vi "test-swerve-drve-odometry-03.vi"() -> (3 "Test Passed":bool)   [LabVIEW 2019]
uses:
  <vilib>/Rock Robotics/WPI/ThirdParty/JAS_Junk/TrajLib/TypeDef/SWERVE_DRIVE_ODOMETRY.ctl
  <vilib>/Rock Robotics/WPI/ThirdParty/JAS_Junk/TrajLib/TypeDef/POSE2D.ctl
  <vilib>/Rock Robotics/WPI/ThirdParty/JAS_Junk/TrajLib/TypeDef/TRANSLATION2D.ctl
  <vilib>/Rock Robotics/WPI/ThirdParty/JAS_Junk/TrajLib/TypeDef/ROTATION2D.ctl
  <vilib>/Rock Robotics/WPI/ThirdParty/JAS_Junk/TrajLib/TypeDef/SWERVE_DRIVE_MODULE_POSITION.ctl
  <vilib>/Rock Robotics/WPI/ThirdParty/JAS_Junk/TrajLib/TypeDef/SWERVE_DRIVE_KINEMATICS.ctl
  <vilib>/Analysis/Matrix/Datatypes/RealMatrix.ctl
  <vilib>/Rock Robotics/WPI/ThirdParty/JAS_Junk/TrajLib/TypeDef/SWERVE_DRIVE_MODULE_STATE.ctl
  <vilib>/Rock Robotics/WPI/ThirdParty/JAS_Junk/TrajLib/Conv_Deg_Radians.vi
  <vilib>/Rock Robotics/WPI/ThirdParty/JAS_Junk/TrajLib/Rotation2d_CreateAngle.vi
  <vilib>/Rock Robotics/WPI/ThirdParty/JAS_Junk/TrajLib/Trajectory_Library.lvlib
  <vilib>/Analysis/Matrix/NI_Matrix.lvlib
panel:
  out "SWERVE_DRIVE_KINEMATICS":T1 {"SavedModuleStates"."Angle"."SIN" format="%13.4f"; "SavedModuleStates"."Angle"."COS" format="%13.4f"; "SavedModuleStates"."Angle"."VALUE" format="%13.4f"; "PrevCoR"."Y" format="%14.3f"; "PrevCoR"."X" format="%14.3f"; "Modules"."Y" format="%14.3f"; "Modules"."X" format="%14.3f"}
  out "robot POSE 3":T6={"TRANSLATION"={"X"=0.0, "Y"=0.0}, "ROTATION"={"VALUE"=0.0, "COS"=1.0, "SIN"=0.0}} {"ROTATION"."SIN" format="%13.4f"; "ROTATION"."COS" format="%13.4f"; "ROTATION"."VALUE" format="%13.4f"; "TRANSLATION"."Y" format="%14.3f"; "TRANSLATION"."X" format="%14.3f"}
  out "Odom 3":T7={"POSE"={"TRANSLATION"={"X"=0.0, "Y"=0.0}, "ROTATION"={"VALUE"=0.0, "COS"=1.0, "SIN"=0.0}}, "GyroOffset"={"VALUE"=0.0, "COS"=1.0, "SIN"=0.0}, "PreviousAngle"={"VALUE"=0.0, "COS"=1.0, "SIN"=0.0}, "PrevModulePositions"=[], "NumModules"=0} {"PrevModulePositions"."Angle"."SIN" format="%13.4f"; "PrevModulePositions"."Angle"."COS" format="%13.4f"; "PrevModulePositions"."Angle"."VALUE" format="%13.4f"; "PreviousAngle"."SIN" format="%13.4f"; "PreviousAngle"."COS" format="%13.4f"; "PreviousAngle"."VALUE" format="%13.4f"; "GyroOffset"."SIN" format="%13.4f"; "GyroOffset"."COS" format="%13.4f"; "GyroOffset"."VALUE" format="%13.4f"; "POSE"."ROTATION"."SIN" format="%13.4f"; "POSE"."ROTATION"."COS" format="%13.4f"; "POSE"."ROTATION"."VALUE" format="%13.4f"; "POSE"."TRANSLATION"."Y" format="%14.3f"; "POSE"."TRANSLATION"."X" format="%14.3f"}
  out "Odom 1":T7={"POSE"={"TRANSLATION"={"X"=0.0, "Y"=0.0}, "ROTATION"={"VALUE"=0.0, "COS"=1.0, "SIN"=0.0}}, "GyroOffset"={"VALUE"=0.0, "COS"=1.0, "SIN"=0.0}, "PreviousAngle"={"VALUE"=0.0, "COS"=1.0, "SIN"=0.0}, "PrevModulePositions"=[], "NumModules"=0} {"PrevModulePositions"."Angle"."SIN" format="%13.4f"; "PrevModulePositions"."Angle"."COS" format="%13.4f"; "PrevModulePositions"."Angle"."VALUE" format="%13.4f"; "PreviousAngle"."SIN" format="%13.4f"; "PreviousAngle"."COS" format="%13.4f"; "PreviousAngle"."VALUE" format="%13.4f"; "GyroOffset"."SIN" format="%13.4f"; "GyroOffset"."COS" format="%13.4f"; "GyroOffset"."VALUE" format="%13.4f"; "POSE"."ROTATION"."SIN" format="%13.4f"; "POSE"."ROTATION"."COS" format="%13.4f"; "POSE"."ROTATION"."VALUE" format="%13.4f"; "POSE"."TRANSLATION"."Y" format="%14.3f"; "POSE"."TRANSLATION"."X" format="%14.3f"}
  out "Odom 0":T7={"POSE"={"TRANSLATION"={"X"=0.0, "Y"=0.0}, "ROTATION"={"VALUE"=0.0, "COS"=1.0, "SIN"=0.0}}, "GyroOffset"={"VALUE"=0.0, "COS"=1.0, "SIN"=0.0}, "PreviousAngle"={"VALUE"=0.0, "COS"=1.0, "SIN"=0.0}, "PrevModulePositions"=[], "NumModules"=0} {"PrevModulePositions"."Angle"."SIN" format="%13.4f"; "PrevModulePositions"."Angle"."COS" format="%13.4f"; "PrevModulePositions"."Angle"."VALUE" format="%13.4f"; "PreviousAngle"."SIN" format="%13.4f"; "PreviousAngle"."COS" format="%13.4f"; "PreviousAngle"."VALUE" format="%13.4f"; "GyroOffset"."SIN" format="%13.4f"; "GyroOffset"."COS" format="%13.4f"; "GyroOffset"."VALUE" format="%13.4f"; "POSE"."ROTATION"."SIN" format="%13.4f"; "POSE"."ROTATION"."COS" format="%13.4f"; "POSE"."ROTATION"."VALUE" format="%13.4f"; "POSE"."TRANSLATION"."Y" format="%14.3f"; "POSE"."TRANSLATION"."X" format="%14.3f"}
  out "robot POSE 0":T6={"TRANSLATION"={"X"=0.0, "Y"=0.0}, "ROTATION"={"VALUE"=0.0, "COS"=1.0, "SIN"=0.0}} {"ROTATION"."SIN" format="%13.4f"; "ROTATION"."COS" format="%13.4f"; "ROTATION"."VALUE" format="%13.4f"; "TRANSLATION"."Y" format="%14.3f"; "TRANSLATION"."X" format="%14.3f"}
  out "robot POSE 2":T6={"TRANSLATION"={"X"=0.0, "Y"=0.0}, "ROTATION"={"VALUE"=0.0, "COS"=1.0, "SIN"=0.0}} {"ROTATION"."SIN" format="%13.4f"; "ROTATION"."COS" format="%13.4f"; "ROTATION"."VALUE" format="%13.4f"; "TRANSLATION"."Y" format="%14.3f"; "TRANSLATION"."X" format="%14.3f"}
  out "Odom 2":T7={"POSE"={"TRANSLATION"={"X"=0.0, "Y"=0.0}, "ROTATION"={"VALUE"=0.0, "COS"=1.0, "SIN"=0.0}}, "GyroOffset"={"VALUE"=0.0, "COS"=1.0, "SIN"=0.0}, "PreviousAngle"={"VALUE"=0.0, "COS"=1.0, "SIN"=0.0}, "PrevModulePositions"=[], "NumModules"=0} {"PrevModulePositions"."Angle"."SIN" format="%13.4f"; "PrevModulePositions"."Angle"."COS" format="%13.4f"; "PrevModulePositions"."Angle"."VALUE" format="%13.4f"; "PreviousAngle"."SIN" format="%13.4f"; "PreviousAngle"."COS" format="%13.4f"; "PreviousAngle"."VALUE" format="%13.4f"; "GyroOffset"."SIN" format="%13.4f"; "GyroOffset"."COS" format="%13.4f"; "GyroOffset"."VALUE" format="%13.4f"; "POSE"."ROTATION"."SIN" format="%13.4f"; "POSE"."ROTATION"."COS" format="%13.4f"; "POSE"."ROTATION"."VALUE" format="%13.4f"; "POSE"."TRANSLATION"."Y" format="%14.3f"; "POSE"."TRANSLATION"."X" format="%14.3f"}
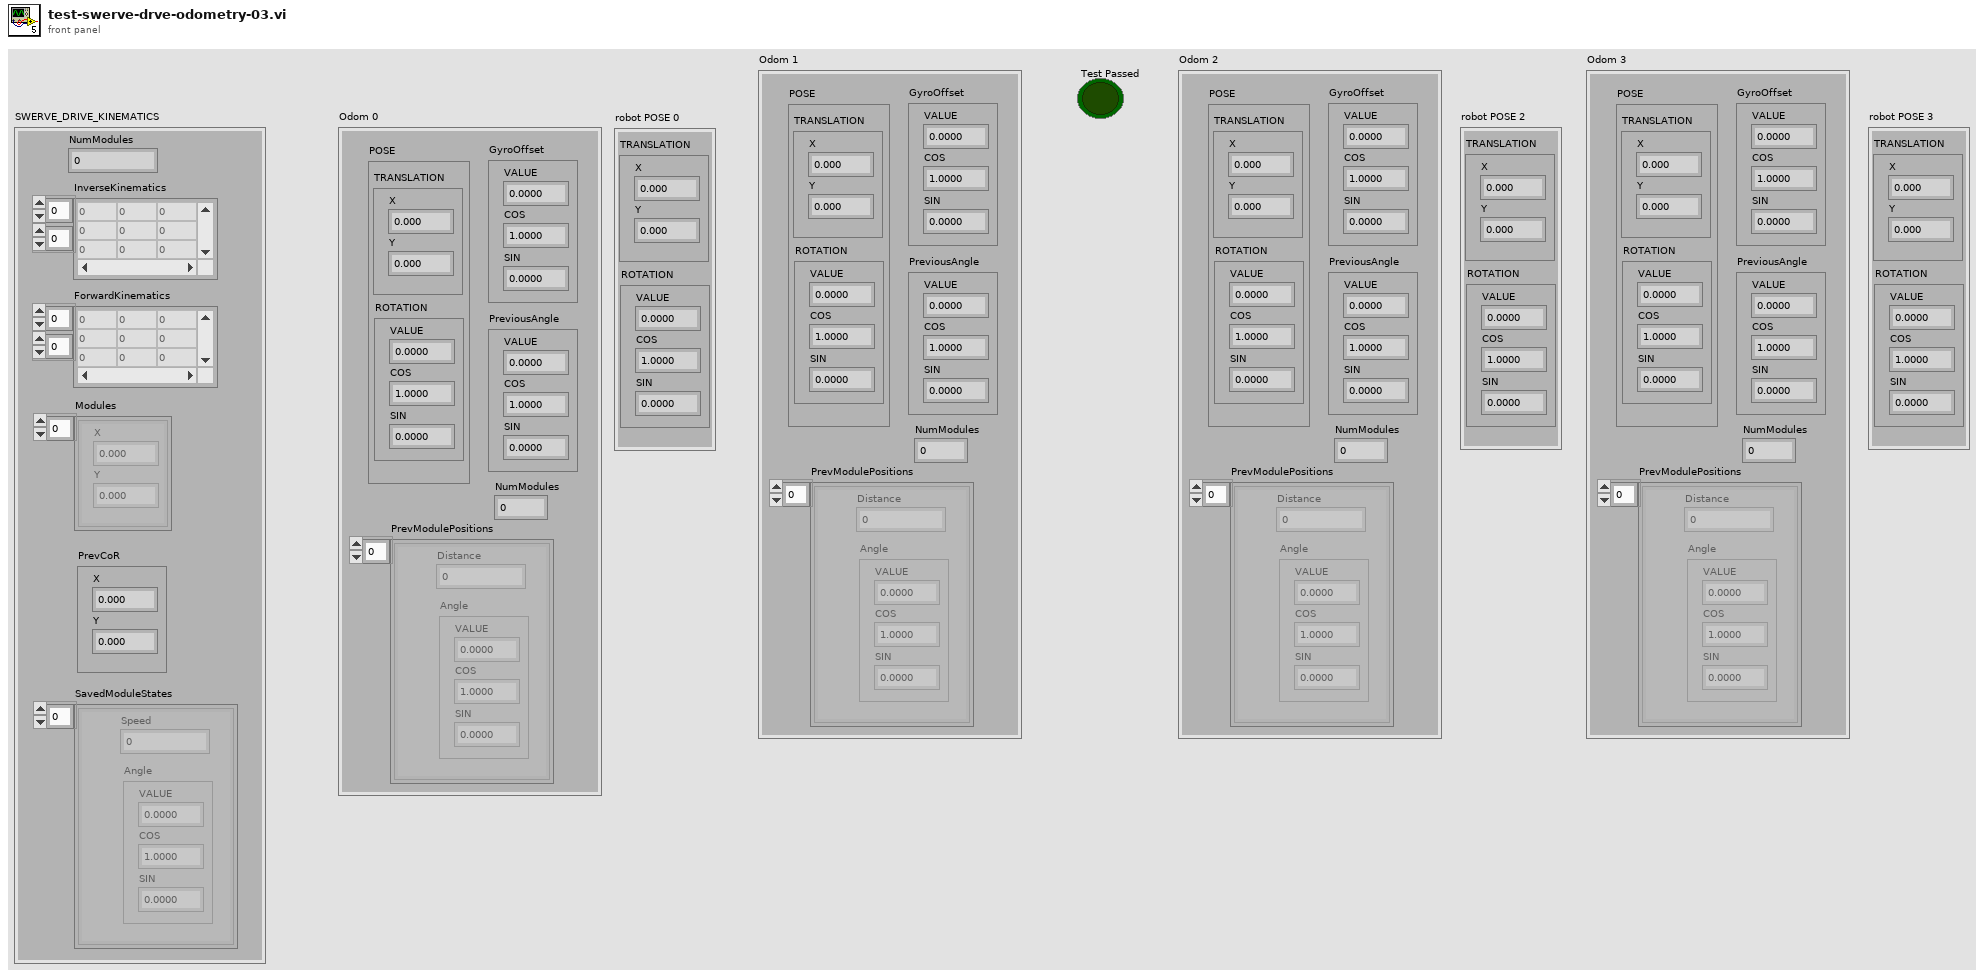
[diagram p1: front panel]
types:
  T1 = typedef "Trajectory_Library.lvlib/SWERVE_DRIVE_KINEMATICS.ctl" = cluster{"NumModules":i32, "InverseKinematics":T2, "ForwardKinematics":T2, "Modules":T3[], "PrevCoR":T3, "SavedModuleStates":T4[]}
  T2 = typedef "NI_Matrix.lvlib/RealMatrix.ctl" = dbl[][]
  T3 = typedef "Trajectory_Library.lvlib/TRANSLATION2D.ctl" = cluster{"X":dbl, "Y":dbl}
  T4 = typedef "Trajectory_Library.lvlib/SWERVE_DRIVE_MODULE_STATE.ctl" = cluster{"Speed":dbl, "Angle":T5}
  T5 = typedef "Trajectory_Library.lvlib/ROTATION2D.ctl" = cluster{"VALUE":dbl, "COS":dbl, "SIN":dbl}
  T6 = typedef "Trajectory_Library.lvlib/POSE2D.ctl" = cluster{"TRANSLATION":T3, "ROTATION":T5}
  T7 = typedef "Trajectory_Library.lvlib/SWERVE_DRIVE_ODOMETRY.ctl" = cluster{"POSE":T6, "GyroOffset":T5, "PreviousAngle":T5, "PrevModulePositions":T8[], "NumModules":i32}
  T8 = typedef "Trajectory_Library.lvlib/SWERVE_DRIVE_MODULE_POSITION.ctl" = cluster{"Distance":dbl, "Angle":T5}
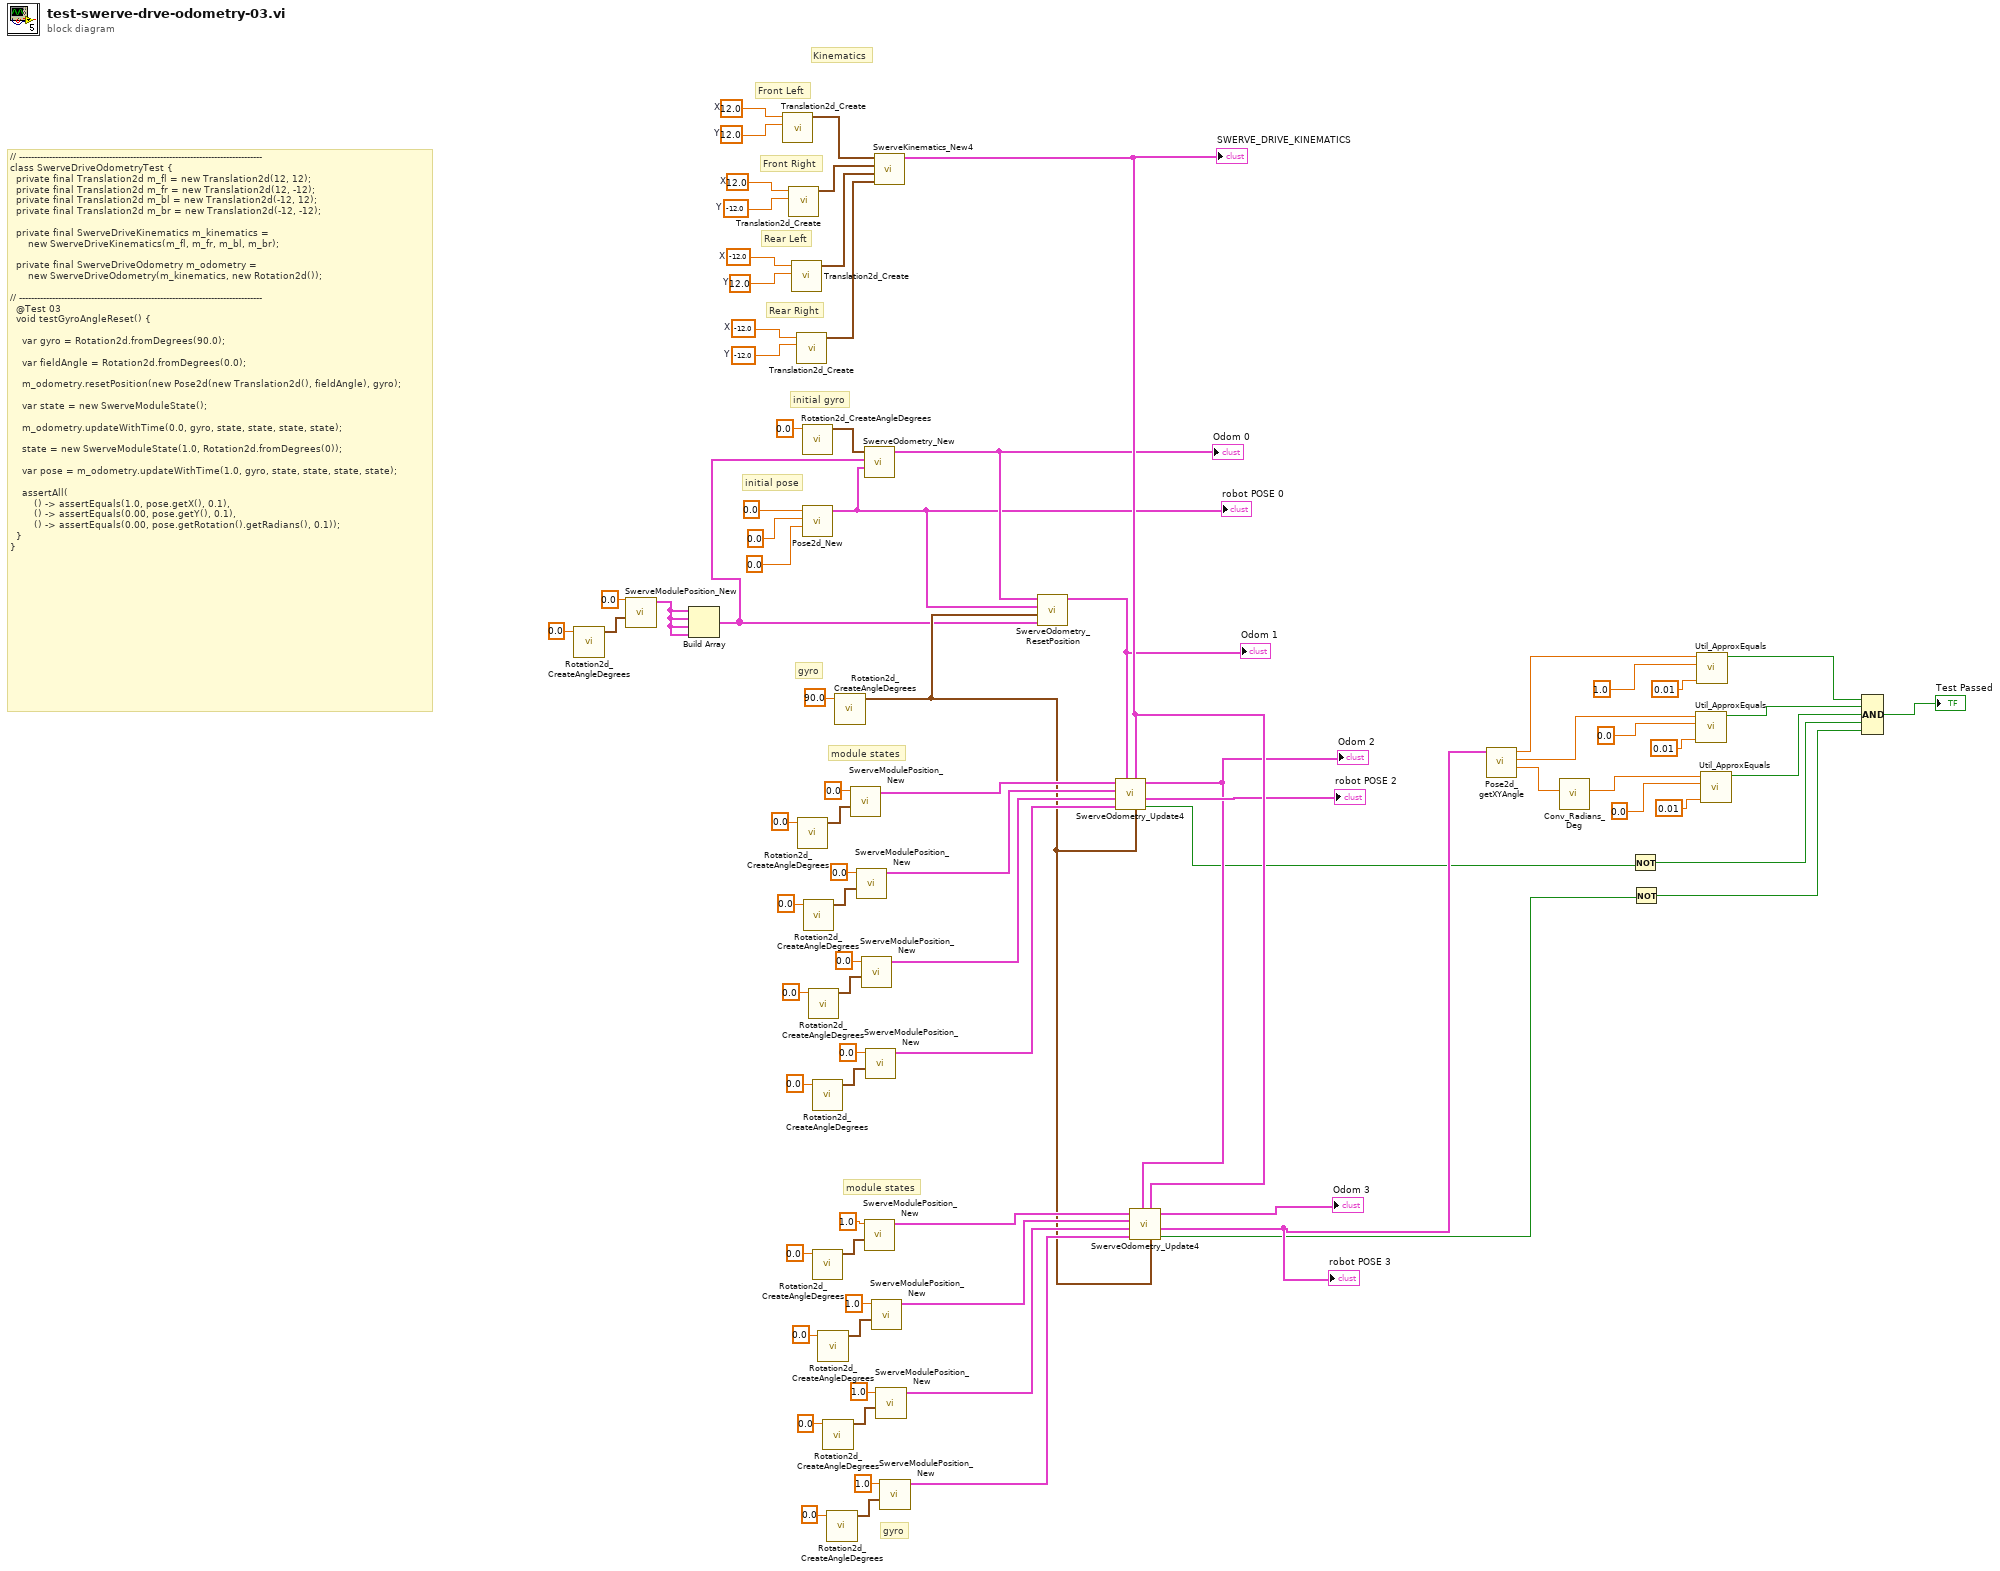
[diagram p0: block diagram]
diagram:
  w78 = -12.0  # X
  w77 = -12.0  # Y
  w76 = -12.0  # X
  w75 = 12.0  # Y
  w74 = 12.0  # X
  w73 = -12.0  # Y
  w72 = 12.0  # X
  w71 = 12.0  # Y
  # "gyro"
  # "initial pose"
  # "gyro"
  # "module states"
  # "module states"
  # "Kinematics"
  # "initial gyro"
  # "Rear Right"
  # "Rear Left"
  # "Front Right"
  # "Front Left"
  # "// ---------------------------------------------------------------------------------\nclass SwerveDriveOdometryTest {\n  private final Translation2d m_fl = new Translation2d(12, 12);\n  private final Translation2d m_fr = new Translation2d(12, -12);\n  private final Translation2d m_bl = new Translation2d(-12, 12);\n  private final Translation2d m_br = new Translation2d(-12, -12);\n\n  private final SwerveDriveKinematics m_kinematics =\n      new SwerveDriveKinematics(m_fl, m_fr, m_bl, m_br);\n\n  private final SwerveDriveOdometry m_odometry =\n      new SwerveDriveOdometry(m_kinematics, new Rotation2d());\n\n// ---------------------------------------------------------------------------------\n  @Test 03\n  void testGyroAngleReset() {\n\n    var gyro = Rotation2d.fromDegrees(90.0);\n\n    var fieldAngle = Rotation2d.fromDegrees(0.0);\n\n    m_odometry.resetPosition(new Pose2d(new Translation2d(), fieldAngle), gyro);\n\n    var state = new SwerveModuleState();\n\n    m_odometry.updateWithTime(0.0, gyro, state, state, state, state);\n\n    state = new SwerveModuleState(1.0, Rotation2d.fromDegrees(0));\n\n    var pose = m_odometry.updateWithTime(1.0, gyro, state, state, state, state);\n\n    assertAll(\n        () -> assertEquals(1.0, pose.getX(), 0.1),\n        () -> assertEquals(0.00, pose.getY(), 0.1),\n        () -> assertEquals(0.00, pose.getRotation().getRadians(), 0.1));\n  }\n}"
  n1 = call <vilib>:"Rotation2d_CreateAngleDegrees.vi"("Angle_Degrees"=0.0) -> ("ROTATION"=w8:T5)  [unwired: 10 in]
  n2 = call <vilib>:"SwerveModulePosition_New.vi"("ROTATION"=w8, "Distance"=0.0 ("Speed")) -> ("SWERVE_DRIVE_MODULE_POSITION"=w6:T8)  [unwired: 9 in]
  n3 = Build Array(w6, w6, w6, w6) -> (w5:T8[])
  n4 = call <vilib>:"Translation2d_Create.vi"("Y"=w71, "X"=w72) -> ("TRANSLATION"=w79:T3)  [unwired: 9 in]
  n5 = call <vilib>:"Translation2d_Create.vi"("Y"=w73, "X"=w74) -> ("TRANSLATION"=w80:T3)  [unwired: 9 in]
  n6 = call <vilib>:"Translation2d_Create.vi"("Y"=w75, "X"=w76) -> ("TRANSLATION"=w81:T3)  [unwired: 9 in]
  n7 = call <vilib>:"Translation2d_Create.vi"("Y"=w77, "X"=w78) -> ("TRANSLATION"=w82:T3)  [unwired: 9 in]
  n8 = call <vilib>:"Rotation2d_CreateAngleDegrees.vi"("Angle_Degrees"=0.0) -> ("ROTATION"=w64:T5)  [unwired: 10 in]
  n9 = call <vilib>:"Rotation2d_CreateAngleDegrees.vi"("Angle_Degrees"=0.0) -> ("ROTATION"=w67:T5)  [unwired: 10 in]
  n10 = call <vilib>:"Pose2d_New.vi"("Heading"=0.0, "Y"=0.0, "X"=0.0) -> ("out POSe"=w13:T6)  [unwired: 8 in]
  "robot POSE 0" <- w13
  n11 = call <vilib>:"Rotation2d_CreateAngleDegrees.vi"("Angle_Degrees"=0.0) -> ("ROTATION"=w61:T5)  [unwired: 10 in]
  n12 = call <vilib>:"Rotation2d_CreateAngleDegrees.vi"("Angle_Degrees"=0.0) -> ("ROTATION"=w58:T5)  [unwired: 10 in]
  n13 = call <vilib>:"Rotation2d_CreateAngleDegrees.vi"("Angle_Degrees"=0.0) -> ("ROTATION"=w55:T5)  [unwired: 10 in]
  n14 = call <vilib>:"Rotation2d_CreateAngleDegrees.vi"("Angle_Degrees"=0.0) -> ("ROTATION"=w48:T5)  [unwired: 10 in]
  n15 = call <vilib>:"Rotation2d_CreateAngleDegrees.vi"("Angle_Degrees"=0.0) -> ("ROTATION"=w45:T5)  [unwired: 10 in]
  n16 = call <vilib>:"Rotation2d_CreateAngleDegrees.vi"("Angle_Degrees"=0.0) -> ("ROTATION"=w42:T5)  [unwired: 10 in]
  n17 = call <vilib>:"Rotation2d_CreateAngleDegrees.vi"("Angle_Degrees"=0.0) -> ("ROTATION"=w39:T5)  [unwired: 10 in]
  n18 = call <vilib>:"Rotation2d_CreateAngleDegrees.vi"("Angle_Degrees"=90.0) -> ("ROTATION"=w12:T5)  [unwired: 10 in]
  n19 = call <vilib>:"SwerveModulePosition_New.vi"("ROTATION"=w64, "Distance"=0.0 ("Speed")) -> ("SWERVE_DRIVE_MODULE_POSITION"=w53:T8)  [unwired: 9 in]
  n20 = call <vilib>:"SwerveModulePosition_New.vi"("ROTATION"=w61, "Distance"=0.0 ("Speed")) -> ("SWERVE_DRIVE_MODULE_POSITION"=w52:T8)  [unwired: 9 in]
  n21 = call <vilib>:"SwerveModulePosition_New.vi"("ROTATION"=w58, "Distance"=0.0 ("Speed")) -> ("SWERVE_DRIVE_MODULE_POSITION"=w51:T8)  [unwired: 9 in]
  n22 = call <vilib>:"SwerveOdometry_New.vi"("InitialPose"=w13, "Module Positions"=w5, "gyroAngle"=w67) -> ("SWERVE_DRIVE_ODOMETRY"=w18:T7)  [unwired: 8 in]
  "Odom 0" <- w18
  n23 = call <vilib>:"SwerveModulePosition_New.vi"("ROTATION"=w48, "Distance"=1.0 ("Speed")) -> ("SWERVE_DRIVE_MODULE_POSITION"=w37:T8)  [unwired: 9 in]
  n24 = call <vilib>:"SwerveModulePosition_New.vi"("ROTATION"=w55, "Distance"=0.0 ("Speed")) -> ("SWERVE_DRIVE_MODULE_POSITION"=w50:T8)  [unwired: 9 in]
  n25 = call <vilib>:"SwerveModulePosition_New.vi"("ROTATION"=w45, "Distance"=1.0 ("Speed")) -> ("SWERVE_DRIVE_MODULE_POSITION"=w36:T8)  [unwired: 9 in]
  n26 = call <vilib>:"SwerveKinematics_New4.vi"("wheel 3"=w82, "wheel 2"=w81, "wheel 1"=w80, "wheel 0"=w79) -> ("SWERVE_DRIVE_KINEMATICS"=w33:T1)  [unwired: 7 in]
  "SWERVE_DRIVE_KINEMATICS" <- w33
  n27 = call <vilib>:"SwerveModulePosition_New.vi"("ROTATION"=w42, "Distance"=1.0 ("Speed")) -> ("SWERVE_DRIVE_MODULE_POSITION"=w35:T8)  [unwired: 9 in]
  n28 = call <vilib>:"SwerveModulePosition_New.vi"("ROTATION"=w39, "Distance"=1.0 ("Speed")) -> ("SWERVE_DRIVE_MODULE_POSITION"=w34:T8)  [unwired: 9 in]
  n29 = call <vilib>:"SwerveOdometry_ResetPosition.vi"("Module Positions"=w5, "gyroAngle"=w12, "Pose"=w13, "in SWERVE_DRIVE_ODOMETRY"=w18) -> ("out SWERVE_DRIVE_ODOMETRY"=w17:T7)  [unwired: 6 in, 1 out]
  "Odom 1" <- w17
  n30 = call <vilib>:"SwerveOdometry_Update4.vi"("gyroAngle"=w12, "SWERVE_DRIVE_KINEMATICS"=w33, "in SWERVE_DRIVE_ODOMETRY"=w17, "Wheel Position 3"=w50, "Wheel Position 2"=w51, "Wheel Position 1"=w52, "Wheel Position 0"=w53) -> ("Error"=w4:bool, "robot POSE"=→"robot POSE 2":T6, "out SWERVE_DRIVE_ODOMETRY"=w15:T7)  [unwired: 2 in]
  "Odom 2" <- w15
  n31 = call <vilib>:"SwerveOdometry_Update4.vi"("gyroAngle"=w12, "SWERVE_DRIVE_KINEMATICS"=w33, "in SWERVE_DRIVE_ODOMETRY"=w15, "Wheel Position 3"=w34, "Wheel Position 2"=w35, "Wheel Position 1"=w36, "Wheel Position 0"=w37) -> ("Error"=w3:bool, "robot POSE"=w10:T6, "out SWERVE_DRIVE_ODOMETRY"=→"Odom 3":T7)  [unwired: 2 in]
  "robot POSE 3" <- w10
  n32 = call <vilib>:"Pose2d_getXYAngle.vi"("in POSE"=w10) -> ("Angle"=w29:dbl, "Y"=w27:dbl, "X"=w28:dbl)  [unwired: 8 in]
  n33 = call <vilib>:"Conv_Radians_Deg.vi"("Radians"=w29) -> ("Degrees"=w26:dbl)  [unwired: 10 in]
  n34 = Not(x=w4) -> (.not. x?=w2:bool)
  n35 = Not(x=w3) -> (.not. x?=w1:bool)
  n36 = call <vilib>:"Util_ApproxEquals.vi"("Tolerance"=0.01, "Value 2"=0.0, "Value 1"=w27) -> ("ApproxEquals"=w21:bool)  [unwired: 8 in]
  n37 = call <vilib>:"Util_ApproxEquals.vi"("Tolerance"=0.01, "Value 2"=1.0, "Value 1"=w28) -> ("ApproxEquals"=w22:bool)  [unwired: 8 in]
  n38 = call <vilib>:"Util_ApproxEquals.vi"("Tolerance"=0.01, "Value 2"=0.0, "Value 1"=w26) -> ("ApproxEquals"=w20:bool)  [unwired: 8 in]
  n39 = Compound Arithmetic op=AND(w22, w21, w20, w2, w1) -> (→"Test Passed":bool)
